vi "Q 1.vi"() -> ()   [LabVIEW 2018]
uses:
  <vilib>/Analysis/5stat.llb/RMS (DBL).vi
  <vilib>/Analysis/baseanly.llb/Mean (DBL).vi
  <vilib>/Analysis/NI_AALBase.lvlib
  <vilib>/Analysis/NI_AALPro.lvlib
panel:
  out "standard deviation":dbl format="%0.2f"
  out "mean":dbl format="%0.2f"
  out "rms value":dbl format="%0.2f"
  out "Root mean square":dbl
  out "Array for root mean square":dbl[](array[numeric])
  out "Mean (second way)":dbl
  out "mean (first way)":dbl format="%0.2f"
  out "Array":dbl[](array[numeric])
  # "Home work 1 \nfirst question"
  # "Mean"
  # "using block of RMS"
  # "standard deviation"
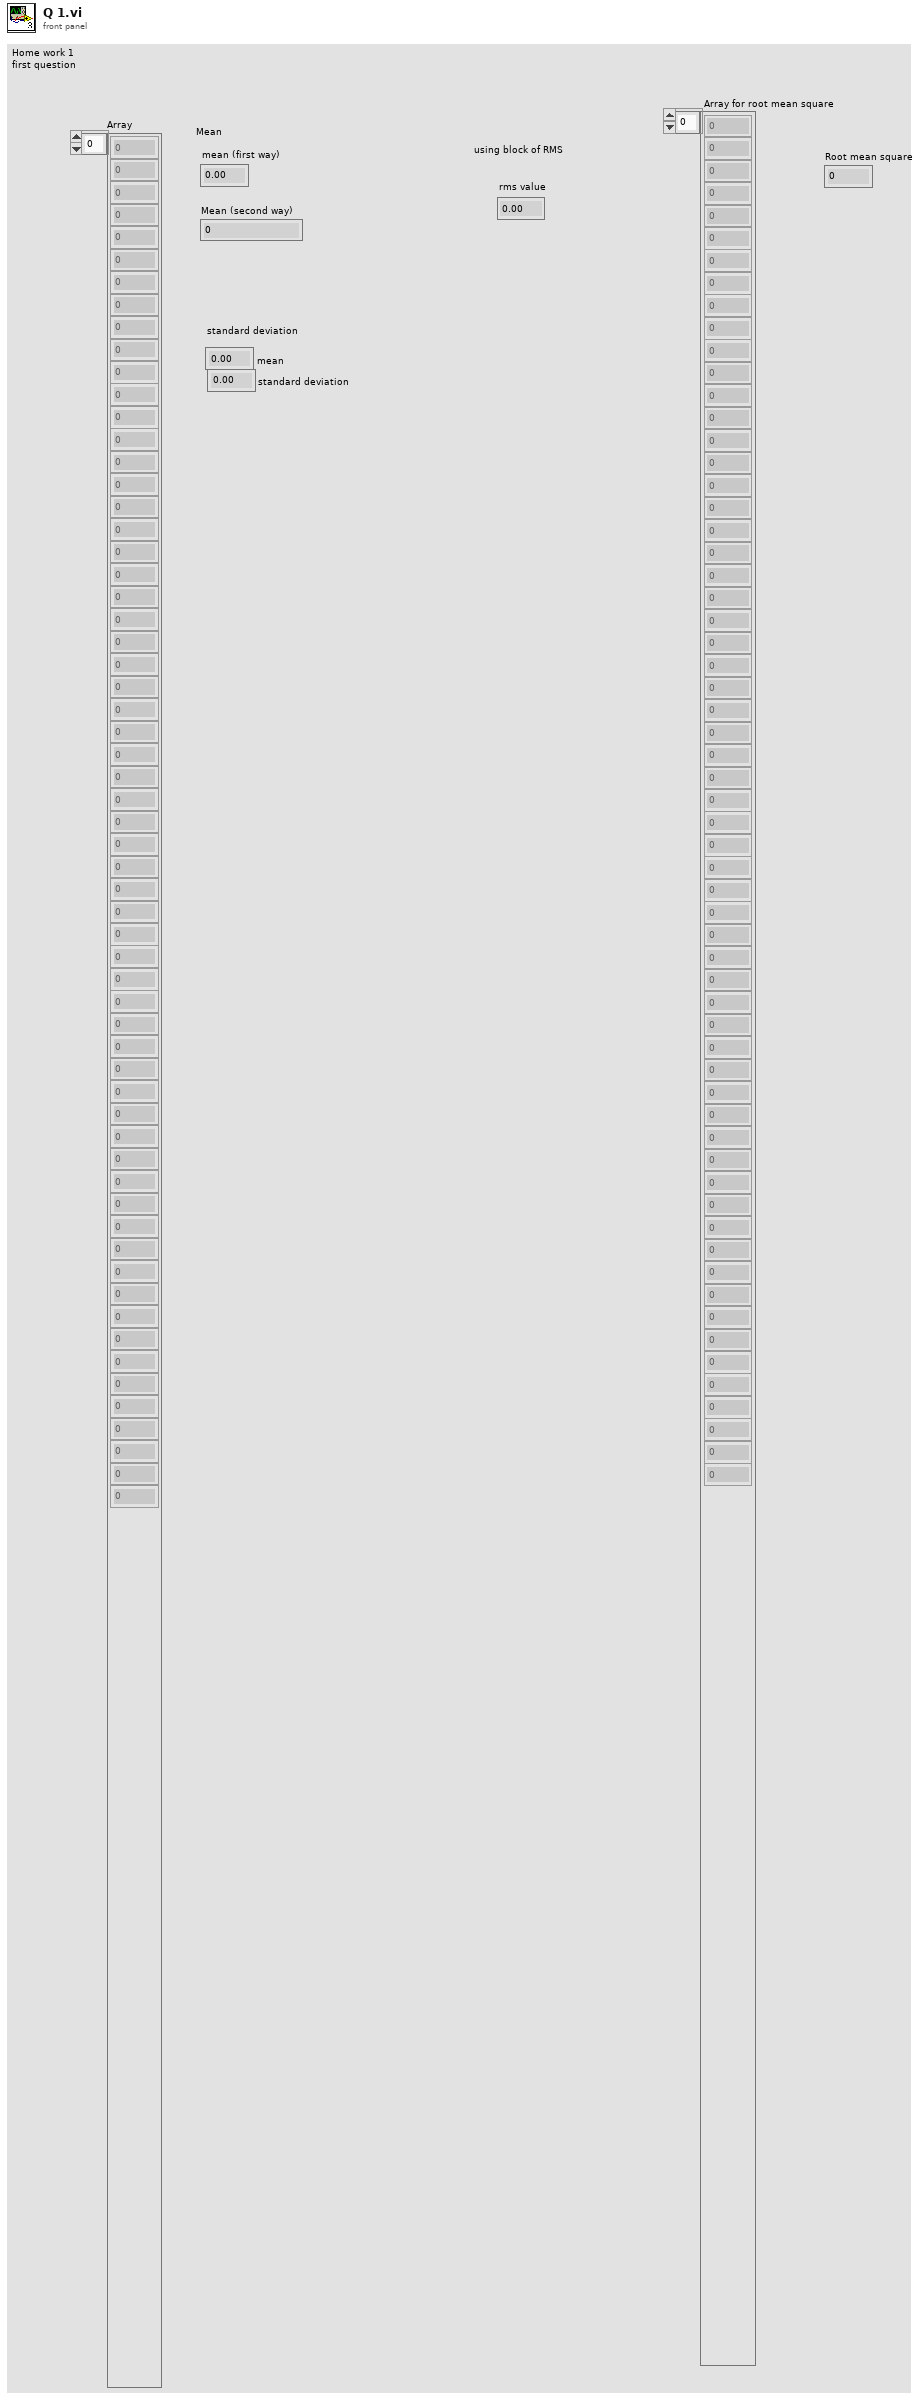
[diagram p1: front panel]
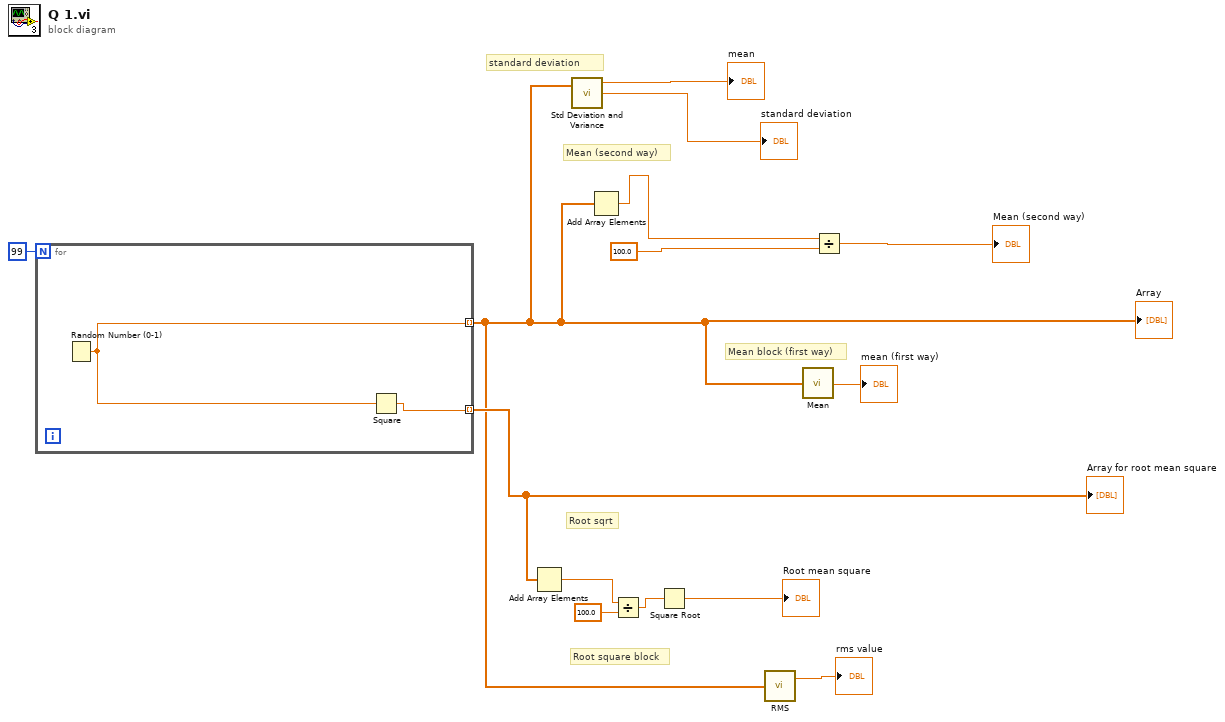
[diagram p0: block diagram]
diagram:
  # "Root square block"
  # "Root sqrt"
  # "Mean (second way)"
  # "Mean block (first way)"
  # "standard deviation"
  n1 = for {
    N: 99 -> [_]
    tunnel: [w16] -> w3 mode=indexing
    tunnel: [w15] -> w5 mode=indexing
    n2 = Random Number (0-1)() -> (number: 0 to 1=w16:dbl)
    n3 = Square(x=w16) -> (x^2=w15:dbl)
  }
  "Array" <- w3
  "Array for root mean square" <- w5
  n4 = Add Array Elements(numeric array=w5) -> (sum=w10:dbl)
  n5 = call <vilib>:"Std Deviation and Variance.vi"("X"=w3) -> ("mean"=→"mean":dbl, "standard deviation"=→"standard deviation":dbl)  [unwired: 1 in, 1 out]
  n6 = Add Array Elements(numeric array=w3) -> (sum=w4:dbl)
  n7 = Divide(x=w10, y=100.0) -> (x/y=w9:dbl)
  n8 = Square Root(x=w9) -> (sqrt(x)=→"Root mean square":dbl)
  n9 = call-poly <vilib>:"RMS.vi"("X"=w3) -> ("rms value"=→"rms value":dbl)  [unwired: 1 out]
  n10 = call-poly <vilib>:"Mean.vi"("X"=w3) -> ("mean"=→"mean (first way)":dbl)  [unwired: 1 out]
  n11 = Divide(x=w4, y=100.0) -> (x/y=→"Mean (second way)":dbl)
